vi "Read Analysis Results.vi"(7 "Channel (1)":i32=1, 8 "error in (no error)":errorcluster, 11 "VISA resource name":refnum<visa-resource-name>) -> (0 "error out":errorcluster, 1 "Stimulus":dbl[](array[numeric]), 2 "Response":dbl[](array[numeric]), 3 "VISA resource name out":refnum<visa-resource-name>, 4 "Number of Analysis Results":i32)   [LabVIEW 2022 SP3, in "Agilent ENA Series.lvlib"]
doc: "Reads out the analysis result of the agena Execute Analysis.vi, for the active trace of selected channel,\n\nNote:\nNumber of analysis result returns for the analysis of the mean value or the search of the maximum value, 1; for the search of all peaks or the search of all targets, the total number of searched measurement points is read out."
uses:
  <instrlib>/Agilent ENA Series/Agilent ENA Series.lvlib
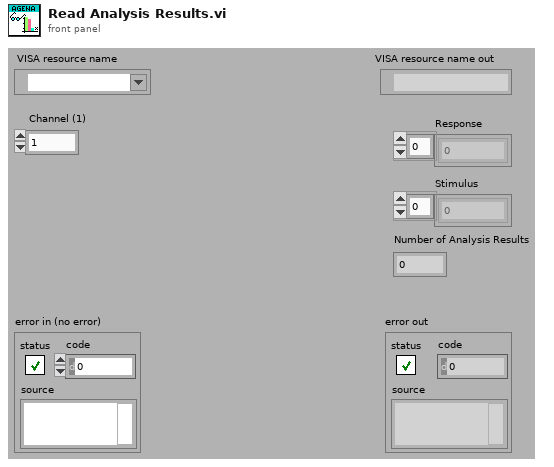
[diagram p1: front panel]
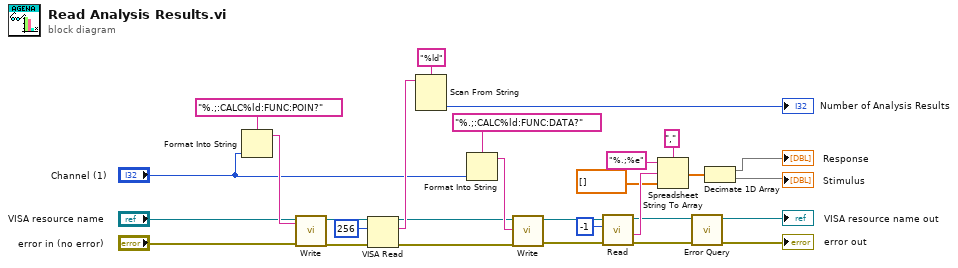
[diagram p0: block diagram]
diagram:
  n1 = Format Into String(format string="%.;:CALC%ld:FUNC:POIN?", "Channel (1)") -> (resulting string=w12:string)  [unwired: 2 in, 1 out]
  n2 = call <instrlib>:"Write.vi"("error in (no error)"="error in (no error)", "String ()"=w12, "VISA resource name"="VISA resource name") -> ("error out"=w10:errorcluster, "VISA resource name out"=w11:refnum<visa-resource-name>)  [unwired: 6 in, 1 out]
  n3 = VISA Read(VISA resource name=w11, byte count=u32 256, error in (no error)=w10) -> (VISA resource name out=w5:refnum<visa-resource-name>, read buffer=w8:string, error out=w4:errorcluster)  [unwired: 1 out]
  n4 = Scan From String(format string="%ld", input string=w8) -> (output 1=→"Number of Analysis Results":i32)  [unwired: 3 in, 3 out]
  n5 = Format Into String(format string="%.;:CALC%ld:FUNC:DATA?", "Channel (1)") -> (resulting string=w28:string)  [unwired: 2 in, 1 out]
  n6 = call <instrlib>:"Write.vi"("error in (no error)"=w4, "String ()"=w28, "VISA resource name"=w5) -> ("error out"=w26:errorcluster, "VISA resource name out"=w27:refnum<visa-resource-name>)  [unwired: 6 in, 1 out]
  n7 = call <instrlib>:"Read.vi"("error in (no error)"=w26, "Number Of Bytes"=-1, "VISA resource name"=w27) -> ("error out"=w16:errorcluster, "String"=w24:string, "VISA resource name out"=w17:refnum<visa-resource-name>)  [unwired: 5 in, 1 out]
  n8 = Spreadsheet String To Array(delimiter (Tab)=",", format string="%.;%e", spreadsheet string=w24, array type (2D Dbl)=dbl[] []) -> (array=w20:dbl[])
  n9 = call <instrlib>:"Error Query.vi"("error in (no error)"=w16, "VISA resource name"=w17) -> ("error out"=→"error out":errorcluster, "VISA resource name out"=→"VISA resource name out":refnum<visa-resource-name>)  [unwired: 6 in, 2 out]
  n10 = Decimate 1D Array(w20) -> (→"Response":dbl[], →"Stimulus":dbl[])
